vi "Calculate PAE.vi"(0 "Amplifier Output Power (dBm)":dbl, 5 "Amplifier Input Power (dBm)":dbl, 7 "Amplifier Vcc":dbl, 9 "Amplifier Icc":dbl) -> (4 "PAE (%)":dbl)   [LabVIEW 2019, in "RDLUtilities.lvlib"]
uses:
  RDLUtilities.lvlib
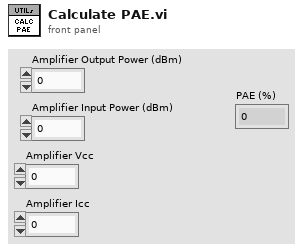
[diagram p1: front panel]
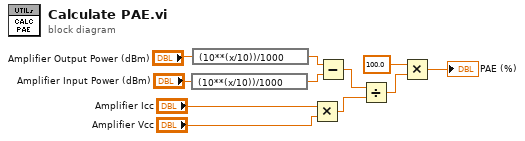
[diagram p0: block diagram]
diagram:
  n1 = expression code="(10**(x/10))/1000"("Amplifier Input Power (dBm)") -> (w2:dbl)
  n2 = expression code="(10**(x/10))/1000"("Amplifier Output Power (dBm)") -> (w1:dbl)
  n3 = Multiply(x="Amplifier Icc", y="Amplifier Vcc") -> (x*y=w9:dbl)
  n4 = Subtract(x=w1, y=w2) -> (x-y=w4:dbl)
  n5 = Divide(x=w4, y=w9) -> (x/y=w8:dbl)
  n6 = Multiply(x=100.0, y=w8) -> (x*y=→"PAE (%)":dbl)
